vi "Set Speed.vi"(8 "error in (no error)":errorcluster, 10 "speed":dbl, 11 "Masterflex Settings in":T1={"VISA resource name"="", "Simulated?"=FALSE, "Pump Number"=1.0, "Reverse?"=FALSE} {"Pump Number" min=1.0 max=20.0 step=1.0}) -> (0 "error out":errorcluster, 1 "Connection Error":bool, 3 "Masterflex Settings out":T1={"VISA resource name"="", "Simulated?"=FALSE, "Pump Number"=1.0, "Reverse?"=FALSE} {"Pump Number" min=1.0 max=20.0 step=1.0})   [LabVIEW 2018, in "Masterflex 7550-30.lvlib"]
uses:
  Masterflex 7550-30.lvlib
  Controls/Settings Cluster.ctl
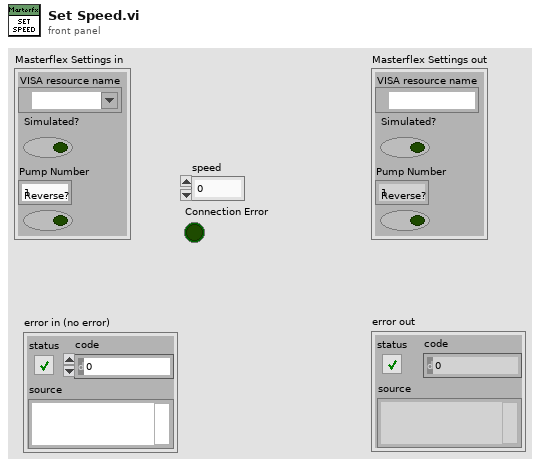
[diagram p1: front panel]
types:
  T1 = typedef "Masterflex 7550-30.lvlib/Settings Cluster.ctl" = cluster{"VISA resource name":refnum<visa-resource-name>, "Simulated?":bool, "Pump Number":dbl, "Reverse?":bool}
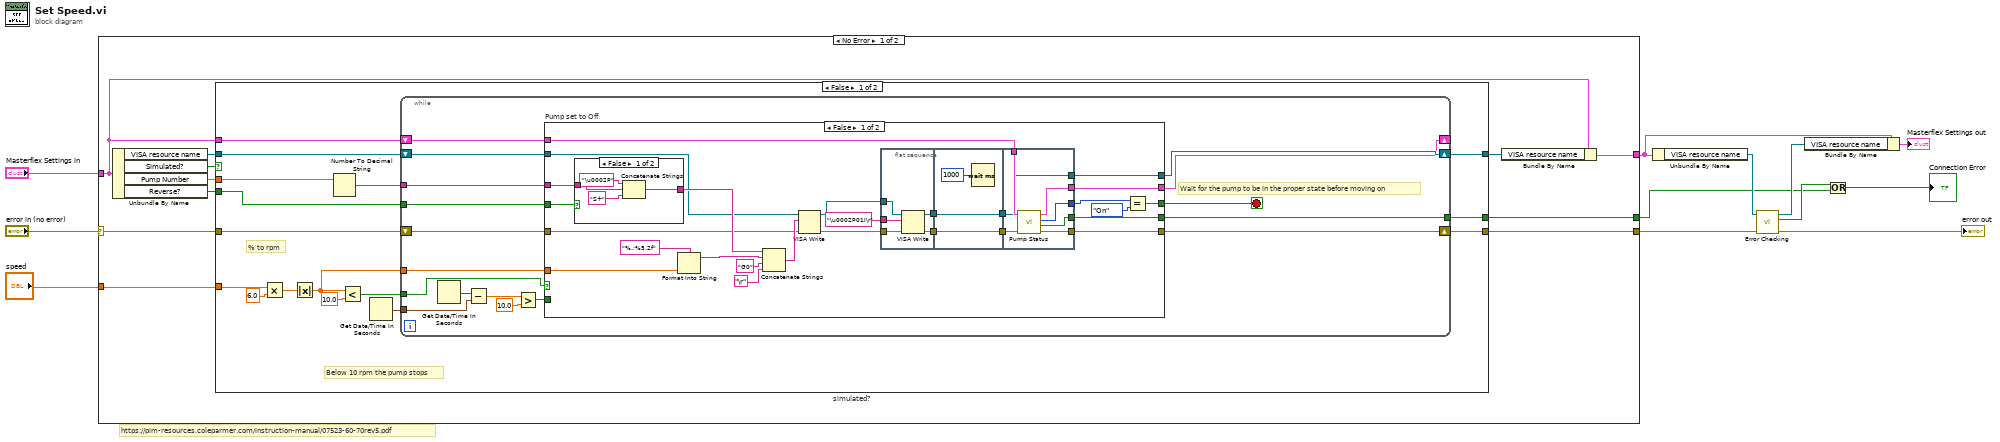
[diagram p0: block diagram]
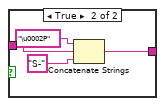
[diagram p2: hidden frame]
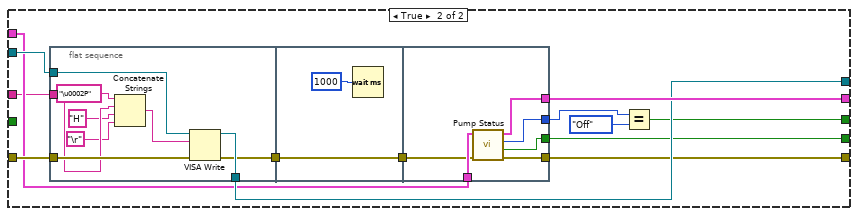
[diagram p3: hidden frame]
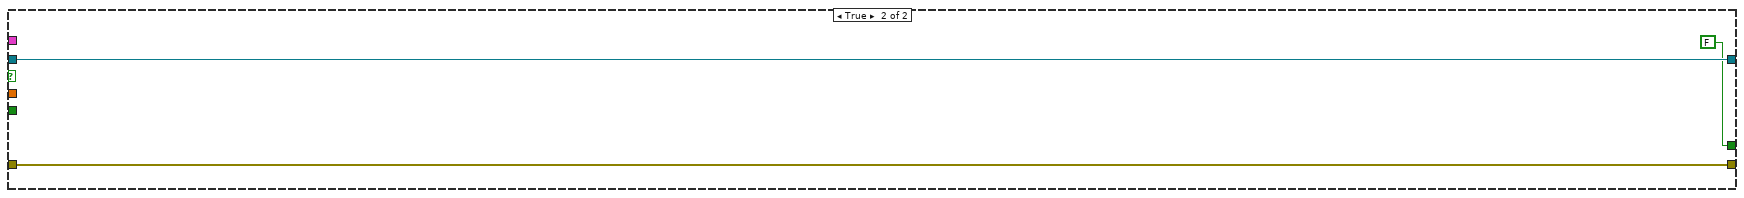
[diagram p4: hidden frame]
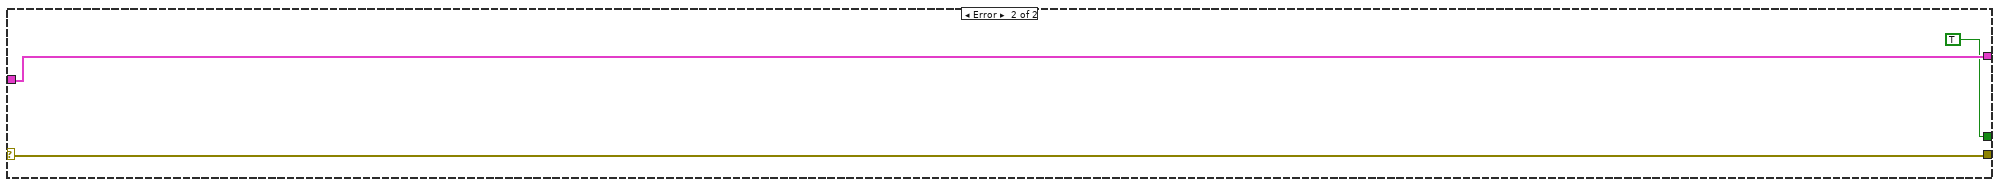
[diagram p5: hidden frame]
diagram:
  # "https://pim-resources.coleparmer.com/instruction-manual/07523-60-70rev5.pdf"
  n1 = case shown="No Error" "error in (no error)" {
    selector: "error in (no error)" -> [w20 w141]
    tunnel: [w19 w141] -> w9
    tunnel: [w17 w140] -> w7
    tunnel: "Masterflex Settings in" -> [w14 w140]
    tunnel: "speed" -> [w18 _]
    tunnel: [w13 TRUE ("Connection Error")] -> w2
    frame No Error {
      n2 = Unbundle By Name(w14) -> ("VISA resource name"=w16:refnum<visa-resource-name>, "Simulated?"=w22:bool, "Pump Number"=w21:dbl, "Reverse?"=w23:bool)
      n3 = case "simulated?" shown="False" w22 {
        tunnel: w20 -> [w30 w138]
        tunnel: [w37 w138] -> w19
        tunnel: w21 -> [w28 _]
        tunnel: w23 -> [w33 _]
        tunnel: w18 -> [w32 _]
        tunnel: w16 -> [w29 w137]
        tunnel: [w31 w137] -> w15
        tunnel: w14 -> [w25 _]
        tunnel: [w24 FALSE ("Connection Error")] -> w13
        frame False {
          # "% to rpm"
          # "Below 10 rpm the pump stops"
          n4 = Multiply(x=w32, y=6.0) -> (x*y=w35:dbl)
          n5 = Absolute Value(x=w35) -> (abs(x)=w34:dbl)
          n6 = Number To Decimal String(number=w28) -> (decimal integer string=w27:string)  [unwired: 1 in]
          n7 = Less?(x=w34, y=10.0) -> (x < y?=w38:bool)
          n8 = Get Date/Time In Seconds() -> (seconds since 1Jan1904=w26:timestamp)
          n9 = while {
            tunnel: w38 -> [w56]
            tunnel: w34 -> [w54]
            tunnel: w33 -> [w53]
            tunnel: w27 -> [w44]
            shift-right: [w55] -> w37
            shift-left: w30 -> [w46]
            shift-right: [w52] -> w31
            shift-left: w29 -> [w45]
            tunnel: w26 -> [w48]
            shift-right: [w47] -> _
            shift-left: w25 -> [w43]
            tunnel: [w42] -> w24
            stop <- w40 stop-if-true
            # "Wait for the pump to be in the proper state before moving on"
            n10 = Get Date/Time In Seconds() -> (seconds since 1Jan1904=w51:timestamp)
            n11 = Subtract(x=w51, y=w48) -> (x-y=w49:dbl)
            n12 = Greater?(x=w49, y=10.0) -> (0:w41:bool)
            n13 = case "Pump set to Off" shown="False" w56 {
              tunnel: [w68 w112] -> w55
              tunnel: w54 -> [w80 _]
              tunnel: w53 -> [w79 _]
              tunnel: [w69 w114] -> w52
              tunnel: w44 -> [w67 w110]
              tunnel: w41 -> [_ _]
              tunnel: w43 -> [w65 w111]
              tunnel: [w64 w117] -> w47
              tunnel: w46 -> [w62 w118]
              tunnel: w45 -> [w63 w113]
              tunnel: [w61 w109] -> w42
              tunnel: [w57 w106] -> w40
              frame False {
                n14 = case shown="False" w79 {
                  tunnel: w67 -> [w100 w103]
                  tunnel: [w98 w102] -> w82
                  frame False {
                    n15 = Concatenate Strings("\u0002P" ("string"), w100, "S+" ("string")) -> (w98:string)
                  }
                  frame True {
                    n16 = Concatenate Strings("\u0002P" ("string"), w103, "S-" ("string")) -> (w102:string)
                  }
                }
                n17 = Format Into String(format string="%.;%5.2f", w80) -> (resulting string=w81:string)  [unwired: 2 in, 1 out]
                n18 = Concatenate Strings(w82, w81, "G0" ("string"), "\r") -> (w77:string)
                n19 = VISA Write(VISA resource name=w63, write buffer=w77, error in (no error)=w62) -> (VISA resource name out=w74:refnum<visa-resource-name>, error out=w76:errorcluster)  [unwired: 1 out]
                n20 = flat-sequence {
                  tunnel: w76 -> [w87]
                  tunnel: "\u0002P01I\r" ("write buffer") -> [w86]
                  tunnel: w74 -> [w85]
                  tunnel: [w84] -> w73
                  tunnel: [w83] -> w70
                  tunnel: w73 -> [w89]
                  tunnel: [w89] -> w72
                  tunnel: [w88] -> w71
                  tunnel: w70 -> [w88]
                  tunnel: w72 -> [w94]
                  tunnel: w71 -> [w96]
                  tunnel: [w94] -> w69
                  tunnel: [w95] -> w68
                  tunnel: w65 -> [w97]
                  tunnel: [w91] -> w64
                  tunnel: [w93] -> w59
                  tunnel: [w92] -> w61
                  frame #0 {
                    n21 = VISA Write(VISA resource name=w85, write buffer=w86, error in (no error)=w87) -> (VISA resource name out=w84:refnum<visa-resource-name>, error out=w83:errorcluster)  [unwired: 1 out]
                  }
                  frame #1 {
                    n22 = Wait (ms)(milliseconds to wait=u32 1000) -> ()  [unwired: 1 out]
                  }
                  frame #2 {
                    n23 = call "Pump Status.vi"("error in (no error)"=w96, "Masterflex Settings in"=w97) -> ("error out"=w95:errorcluster, "Connection Error"=w92:bool, "Pump On?"=w93:enum16{"Off", "On", "Not Initialized"}, "Masterflex Settings out"=w91:T1)  [unwired: 6 in]
                  }
                }
                n24 = Equal?(x=w59, y=enum16{"Off", "On", "Not Initialized"}."On") -> (x = y?=w57:bool)
              }
              frame True {
                n25 = flat-sequence {
                  tunnel: w118 -> [w126]
                  tunnel: w113 -> [w125]
                  tunnel: w110 -> [w123]
                  tunnel: [w120] -> w114
                  tunnel: [w119] -> w115
                  tunnel: [w128] -> w116
                  tunnel: w115 -> [w128]
                  tunnel: w111 -> [w135]
                  tunnel: [w134] -> w108
                  tunnel: [w133] -> w117
                  tunnel: w116 -> [w132]
                  tunnel: [w131] -> w112
                  tunnel: [w130] -> w109
                  frame #0 {
                    n26 = Concatenate Strings("\u0002P" ("string"), w123, "H" ("string"), "\r") -> (w127:string)
                    n27 = VISA Write(VISA resource name=w125, write buffer=w127, error in (no error)=w126) -> (VISA resource name out=w120:refnum<visa-resource-name>, error out=w119:errorcluster)  [unwired: 1 out]
                  }
                  frame #1 {
                    n28 = Wait (ms)(milliseconds to wait=u32 1000) -> ()  [unwired: 1 out]
                  }
                  frame #2 {
                    n29 = call "Pump Status.vi"("error in (no error)"=w132, "Masterflex Settings in"=w135) -> ("error out"=w131:errorcluster, "Connection Error"=w130:bool, "Pump On?"=w134:enum16{"Off", "On", "Not Initialized"}, "Masterflex Settings out"=w133:T1)  [unwired: 6 in]
                  }
                }
                n30 = Equal?(x=w108, y=enum16{"Off", "On", "Not Initialized"}."Off") -> (x = y?=w106:bool)
              }
            }
          }
        }
        frame True {
        }
      }
      n31 = Bundle By Name(cluster=w14, "VISA resource name"=w15) -> (w17:T1)
    }
    frame Error {
    }
  }
  n32 = Unbundle By Name(w7) -> ("VISA resource name"=w12:refnum<visa-resource-name>)
  n33 = call "Error Checking.vi"("error in (no error)"=w9, "VISA resource name"=w12) -> ("error out"=→"error out":errorcluster, "Connection Error"=w3:bool, "VISA resource name"=w11:refnum<visa-resource-name>)  [unwired: 7 in]
  n34 = Bundle By Name(cluster=w7, "VISA resource name"=w11) -> (→"Masterflex Settings out":T1)
  n35 = Or(x=w3, y=w2) -> (x .or. y?=→"Connection Error":bool)
